vi "ConstructorTypeString.vi"(6 "error in":errorcluster, 9 "Terminal in":refnum<class "Terminal.lvclass">) -> (0 "error out":errorcluster, 3 "Terminal out":refnum<class "Terminal.lvclass">, 4 "constructor string":string)   [LabVIEW 2014, in "Raspberry Pi Compatible Compiler for LabVIEW.lvlib" / "Terminal.lvclass"]
uses:
  Terminal.lvclass
  Python/Parsing/Python Functions.lvlib
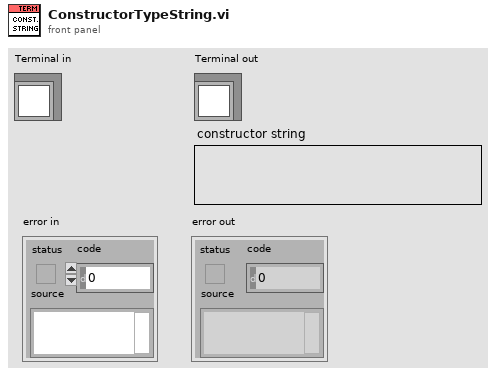
[diagram p1: front panel]
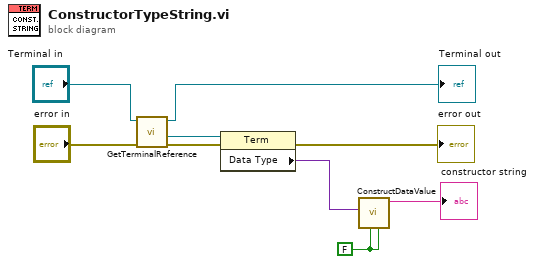
[diagram p0: block diagram]
diagram:
  w7 = FALSE ("value")
  n1 = call "GetTerminalReference.vi"("error in"="error in", "Terminal in"="Terminal in") -> ("error out"=w4:errorcluster, "reference"=w3:refnum<vi>, "Terminal out"=→"Terminal out":refnum<class "Terminal.lvclass">)  [unwired: 7 in]
  n2 = property class="Term"(reference=w3, error in=w4) -> (error out=→"error out":errorcluster, "Data Type"=w6:variant)  [unwired: 1 out]
  n3 = call "ConstructDataValue.vi"("label"=w7, "value"=w7, "Value"=w6) -> ("value"=→"constructor string":string)  [unwired: 5 in, 1 out]
